vi "Parse WMIC Drives.vi"(11 "WMIC Result":string="DeviceID  FreeSpace     Size           \r\r\nC:        142842310656  509722226688   \r\r\nD:        600636674048  2000381014016  \r\r\n\r\r\n") -> (3 "Drives":map{string, T1}(c390))   [LabVIEW 2020, in "Volatus.lvlib" / "Windows System SAL.lvclass"]
uses:
  Windows System SAL.lvclass
  Drive Info.ctl
  <vilib>/Utility/error.llb/whitespace.ctl
  Windows System SAL.lvclass/Windows System SAL.ctl
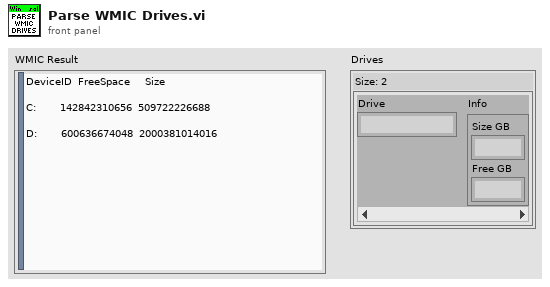
[diagram p1: front panel]
types:
  T1 = typedef "Volatus.lvlib/Windows System SAL.lvclass/Drive Info.ctl" = cluster{"Size GB":dbl, "Free GB":dbl}
  T2 = typedef "whitespace.ctl" = u16
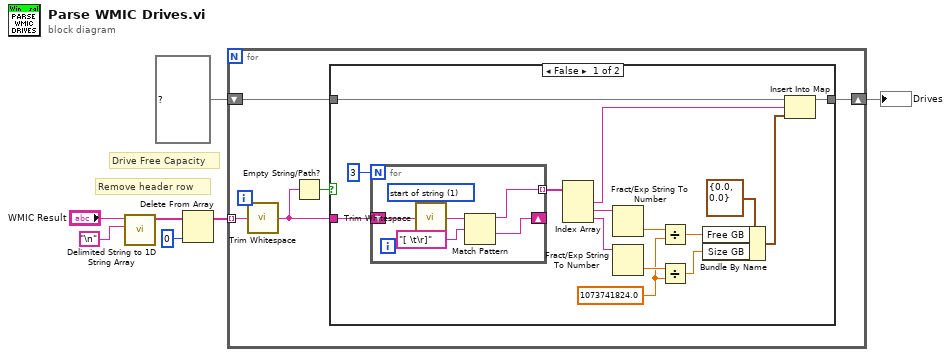
[diagram p0: block diagram]
diagram:
  # "Drive Free Capacity"
  # "Remove header row"
  n1 = call <vilib>:"Delimited String to 1D String Array.vi"("delimiter"="\n", "delimited string"="WMIC Result") -> ("string array"=w4:string[])  [unwired: 9 in]
  n2 = Delete From Array(array=w4, index=0) -> (array with subset deleted=w3:string[])  [unwired: 1 in, 1 out]
  n3 = for {
    tunnel: w3 -> [w10] mode=indexing
    shift-right: [w12] -> w1
    shift-left: map{string, T1} {} ("Map") -> [w11]
    n4 = call <vilib>:"Trim Whitespace.vi"("string"=w10) -> ("trimmed string"=w8:string)  [unwired: 1 in]
    n5 = Empty String/Path?(string/path=w8) -> (empty?=w9:bool)
    n6 = case shown="False" w9 {
      tunnel: [w25 w34] -> w12
      tunnel: w11 -> [w24 w34]
      tunnel: w8 -> [w13 _]
      frame False {
        w17 = 1073741824.0
        n7 = for {
          N: 3 -> [_]
          shift-right: [w28] -> _
          shift-left: w13 -> [w33]
          tunnel: [w29] -> w26 mode=indexing
          w32 = T2 1 items=["both", "start of string", "end of string"] ("location (both)")
          n8 = call <vilib>:"Trim Whitespace.vi"("string"=w33, "location (both)"=w32) -> ("trimmed string"=w31:string)
          n9 = Match Pattern(string=w31, regular expression="[ \t\r]") -> (before substring=w29:string, after substring=w28:string)  [unwired: 1 in, 2 out]
        }
        n10 = Index Array(array=w26) -> (element #1=w23:string, element #2=w20:string, element #3=w21:string)  [unwired: 3 in]
        n11 = Fract/Exp String To Number(string=w20) -> (number=w19:dbl)  [unwired: 3 in, 1 out]
        n12 = Fract/Exp String To Number(string=w21) -> (number=w18:dbl)  [unwired: 3 in, 1 out]
        n13 = Divide(x=w19, y=w17) -> (x/y=w16:dbl)
        n14 = Divide(x=w18, y=w17) -> (x/y=w15:dbl)
        n15 = Bundle By Name(cluster=T1 {"Size GB"=0.0, "Free GB"=0.0} ("Drive Info"), "Free GB"=w16, "Size GB"=w15) -> (w14:T1)
        n16 = Insert Into Map(map in=w24, key=w23, value=w14) -> (map out=w25:map{string, T1})  [unwired: 2 out]
      }
      frame True {
      }
    }
  }
  "Drives" <- w1
